vi "sub UI get Value.vi"(8 "error in":errorcluster, 11 "num ref":refnum<vi>) -> (0 "error out":errorcluster, 1 "valid":bool, 2 "Value":variant)   [LabVIEW 2018, in "LF2R IDE.lvlib" / "LF2R IDE.lvclass"]
uses:
  LF2R IDE.lvclass
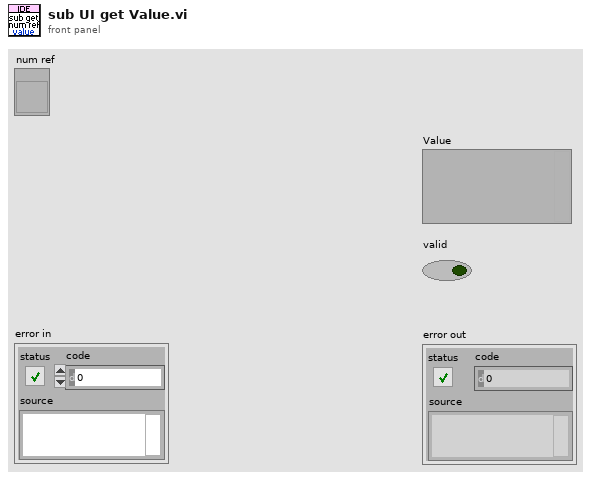
[diagram p1: front panel]
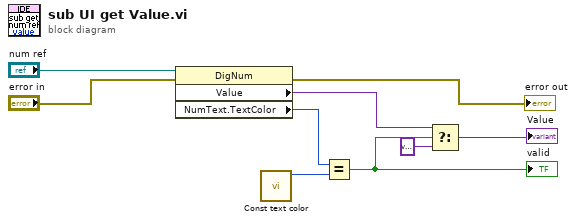
[diagram p0: block diagram]
diagram:
  n1 = property class="DigNum"(reference="num ref", error in="error in") -> (error out=→"error out":errorcluster, "Value"=w3:variant, "NumText.TextColor"=w6:u32)  [unwired: 1 out]
  n2 = call "Const text color.vi"() -> ("valid num color"=w5:u32)  [unwired: 10 in, 1 out]
  n3 = Equal?(x=w6, y=w5) -> (x = y?=w4:bool)
  "valid" <- w4
  n4 = Select(t=w3, s=w4, f=variant) -> (s? t:f=→"Value":variant)
